vi "getFileSystem.vi"(8 "error in (no error)":errorcluster, 10 "computer":string, 11 "FileSystem in":refnum<class "FileSystem.lvclass">) -> (0 "error out":errorcluster, 3 "FileSystem out":refnum<class "FileSystem.lvclass">)   [LabVIEW 2009, in "Tools.lvlib" / "Filing.lvlib" / "FileSystem.lvclass"]
uses:
  FileSystem.lvclass
  FileSystem.lvclass/FileSystem.ctl
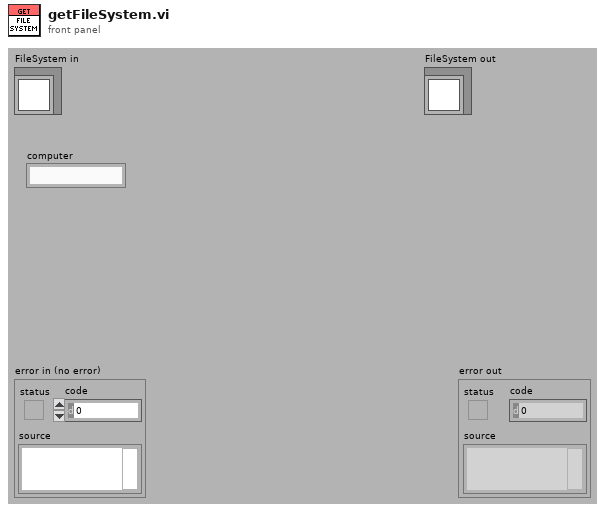
[diagram p1: front panel]
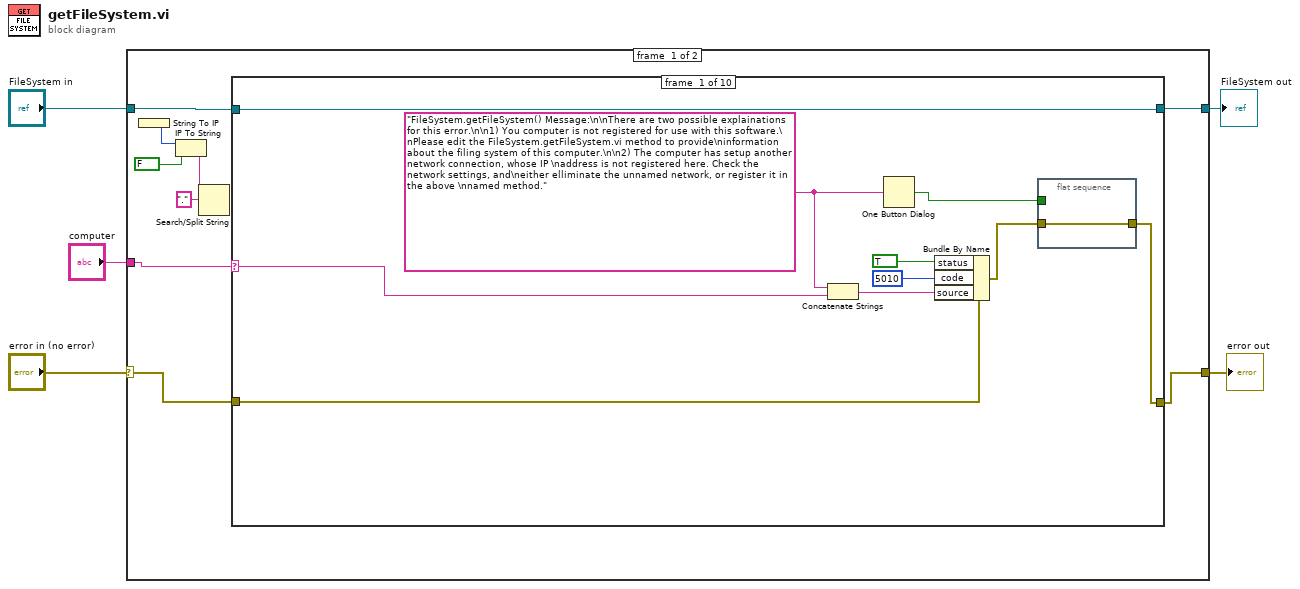
[diagram p0: block diagram]
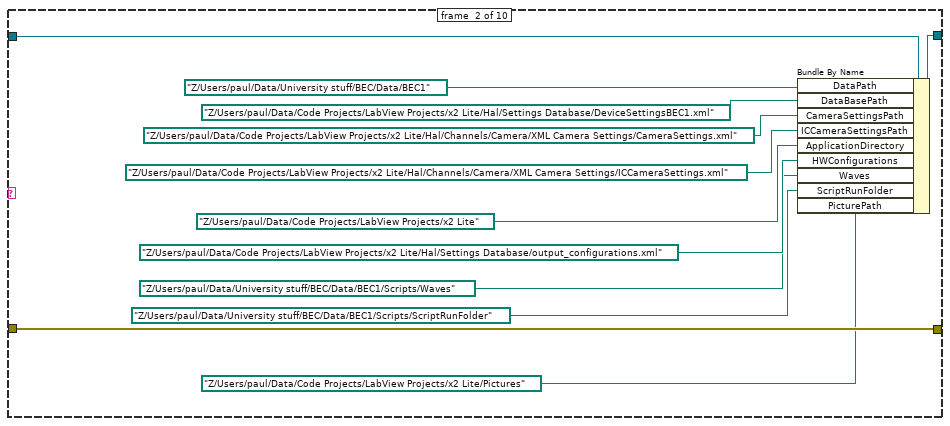
[diagram p2: hidden frame]
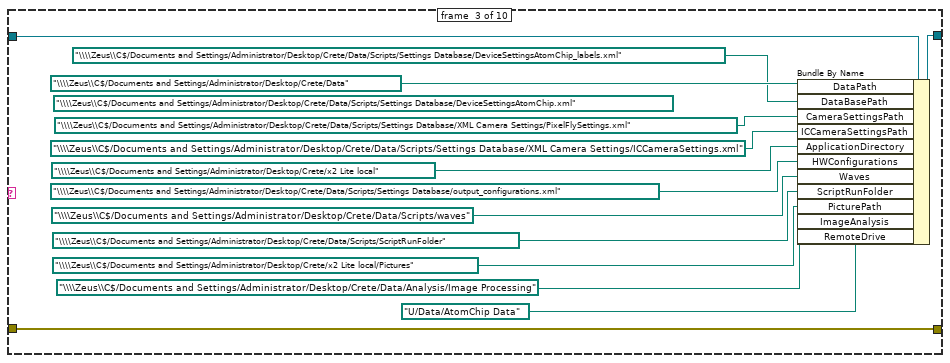
[diagram p3: hidden frame]
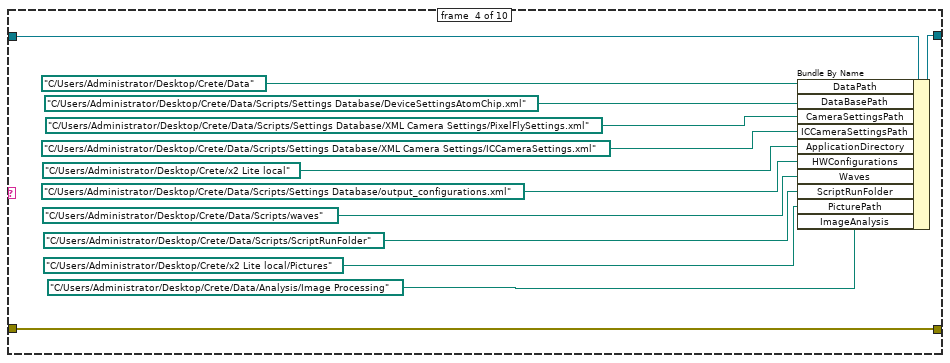
[diagram p4: hidden frame]
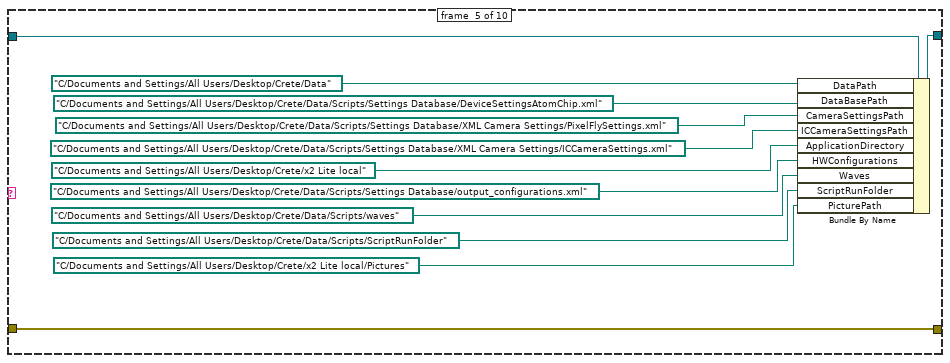
[diagram p5: hidden frame]
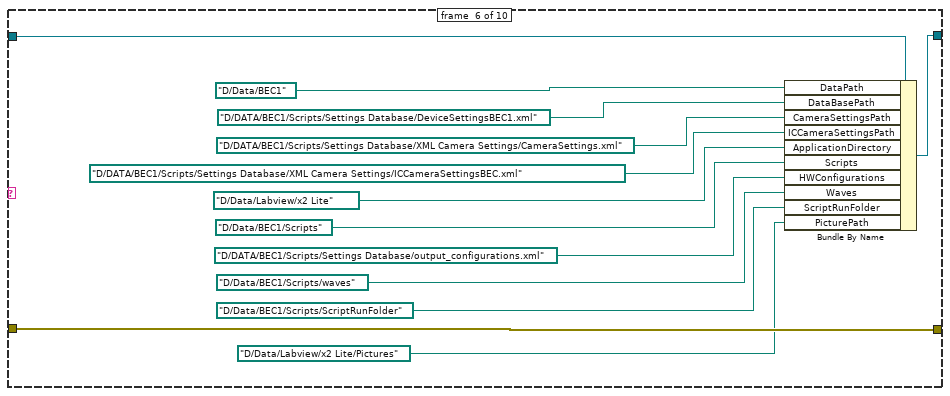
[diagram p6: hidden frame]
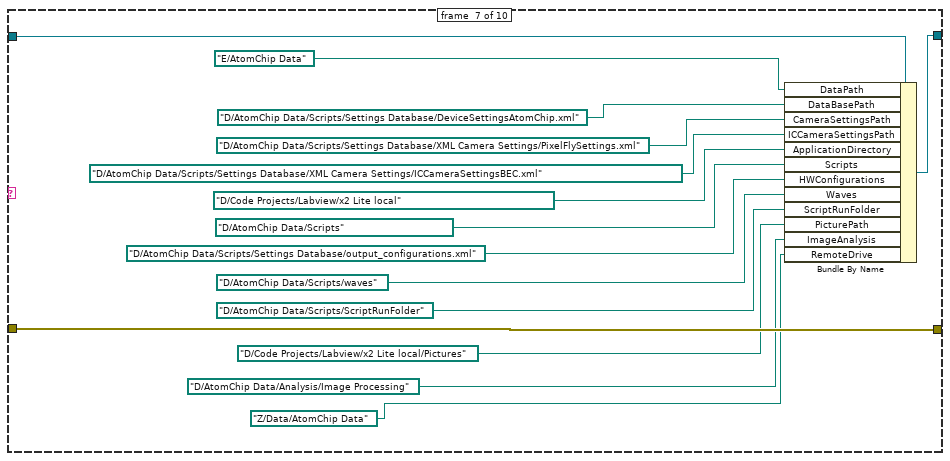
[diagram p7: hidden frame]
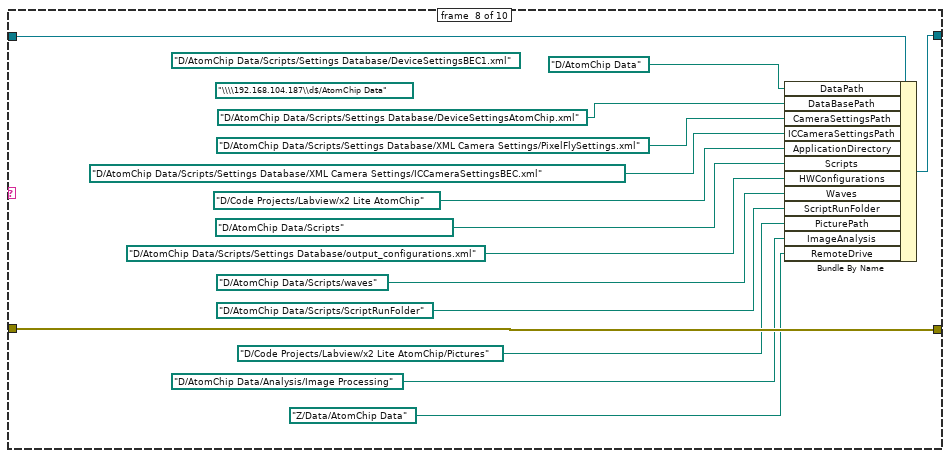
[diagram p8: hidden frame]
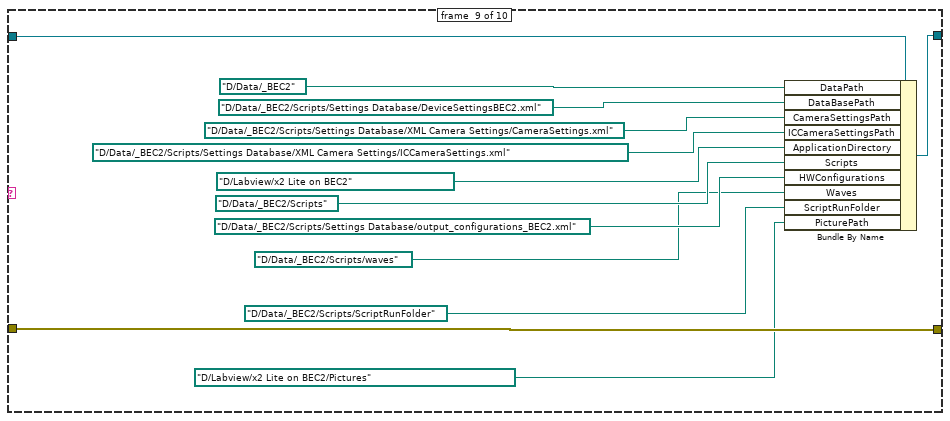
[diagram p9: hidden frame]
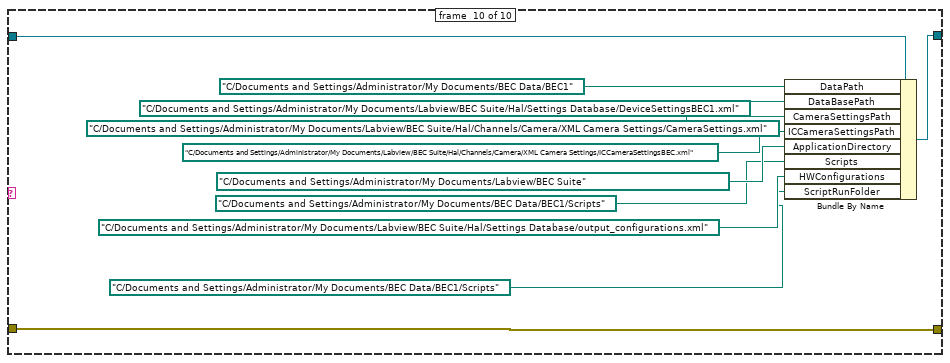
[diagram p10: hidden frame]
diagram:
  n1 = case shown="No Error" "error in (no error)" {
    selector: "error in (no error)" -> [w10 w145]
    tunnel: [w9 w145] -> w4
    tunnel: [w11 w144] -> w2
    tunnel: "FileSystem in" -> [w12 w144]
    tunnel: "computer" -> [w6 _]
    frame #0 {
      n2 = String To IP() -> (0:w13:u32)  [unwired: 1 in]
      n3 = IP To String(1:FALSE, 2:w13) -> (0:w8:string)
      n4 = Search/Split String(string=w8, search string/char (-)=".") -> ()  [unwired: 1 in, 3 out]
      n5 = case shown="\"192.168.104.187\", \"exp1\"" w6 {
        selector: w6 -> [w16 _ _ _ _ _ _ _ _ _]
        tunnel: w12 -> [w24 w37 w51 w64 w76 w89 w104 w119 w132 w143]
        tunnel: [w24 w36 w50 w63 w75 w88 w103 w118 w131 w142] -> w11
        tunnel: w10 -> [w21 w32 w47 w59 w71 w84 w100 w116 w127 w138]
        tunnel: [w19 w32 w47 w59 w71 w84 w100 w116 w127 w138] -> w9
        frame #0 {
          w17 = "FileSystem.getFileSystem() Message:\n\nThere are two possible explainations for this error.\n\n1) You computer is not registered for use with this software.\nPlease edit the FileSystem.getFileSystem.vi method to provide\ninformation about the filing system of this computer.\n\n2) The computer has setup another network connection, whose IP \naddress is not registered here. Check the network settings, and\neither elliminate the unnamed network, or register it in the above \nnamed method."
          n6 = Concatenate Strings(w17, w16) -> (w15:string)
          n7 = One Button Dialog(message=w17) -> (true=w18:bool)  [unwired: 1 in]
          n8 = Bundle By Name(cluster=w21, "status"=TRUE, "code"=5010, "source"=w15) -> (w20:errorcluster)
          n9 = flat-sequence {
            tunnel: w20 -> [w25]
            tunnel: [w25] -> w19
            tunnel: w18 -> [_]
            frame #0 {
            }
          }
        }
        frame #1 {
          n10 = Bundle By Name(cluster=w37, "DataPath"=path "Z:/Users/paul/Data/University stuff/BEC/Data/BEC1", "DataBasePath"=path "Z:/Users/paul/Data/Code Projects/LabView Projects/x2 Lite/Hal/Settings Database/DeviceSettingsBEC1.xml", "CameraSettingsPath"=path "Z:/Users/paul/Data/Code Projects/LabView Projects/x2 Lite/Hal/Channels/Camera/XML Camera Settings/CameraSettings.xml", "ICCameraSettingsPath"=path "Z:/Users/paul/Data/Code Projects/LabView Projects/x2 Lite/Hal/Channels/Camera/XML Camera Settings/ICCameraSettings.xml", "ApplicationDirectory"=path "Z:/Users/paul/Data/Code Projects/LabView Projects/x2 Lite", "HWConfigurations"=path "Z:/Users/paul/Data/Code Projects/LabView Projects/x2 Lite/Hal/Settings Database/output_configurations.xml", "Waves"=path "Z:/Users/paul/Data/University stuff/BEC/Data/BEC1/Scripts/Waves", "ScriptRunFolder"=path "Z:/Users/paul/Data/University stuff/BEC/Data/BEC1/Scripts/ScriptRunFolder", "PicturePath"=path "Z:/Users/paul/Data/Code Projects/LabView Projects/x2 Lite/Pictures") -> (w36:refnum<class "FileSystem.lvclass">)
        }
        frame #2 {
          (unwired) path "\\\\Zeus\\C$/Documents and Settings/Administrator/Desktop/Crete/Data/Scripts/Settings Database/DeviceSettingsAtomChip.xml"
          n11 = Bundle By Name(cluster=w51, "DataPath"=path "\\\\Zeus\\C$/Documents and Settings/Administrator/Desktop/Crete/Data", "DataBasePath"=path "\\\\Zeus\\C$/Documents and Settings/Administrator/Desktop/Crete/Data/Scripts/Settings Database/DeviceSettingsAtomChip_labels.xml", "CameraSettingsPath"=path "\\\\Zeus\\C$/Documents and Settings/Administrator/Desktop/Crete/Data/Scripts/Settings Database/XML Camera Settings/PixelFlySettings.xml", "ICCameraSettingsPath"=path "\\\\Zeus\\C$/Documents and Settings/Administrator/Desktop/Crete/Data/Scripts/Settings Database/XML Camera Settings/ICCameraSettings.xml", "ApplicationDirectory"=path "\\\\Zeus\\C$/Documents and Settings/Administrator/Desktop/Crete/x2 Lite local", "HWConfigurations"=path "\\\\Zeus\\C$/Documents and Settings/Administrator/Desktop/Crete/Data/Scripts/Settings Database/output_configurations.xml", "Waves"=path "\\\\Zeus\\C$/Documents and Settings/Administrator/Desktop/Crete/Data/Scripts/waves", "ScriptRunFolder"=path "\\\\Zeus\\C$/Documents and Settings/Administrator/Desktop/Crete/Data/Scripts/ScriptRunFolder", "PicturePath"=path "\\\\Zeus\\C$/Documents and Settings/Administrator/Desktop/Crete/x2 Lite local/Pictures", "ImageAnalysis"=path "\\\\Zeus\\C$/Documents and Settings/Administrator/Desktop/Crete/Data/Analysis/Image Processing", "RemoteDrive"=path "U:/Data/AtomChip Data") -> (w50:refnum<class "FileSystem.lvclass">)
        }
        frame #3 {
          n12 = Bundle By Name(cluster=w64, "DataPath"=path "C:/Users/Administrator/Desktop/Crete/Data", "DataBasePath"=path "C:/Users/Administrator/Desktop/Crete/Data/Scripts/Settings Database/DeviceSettingsAtomChip.xml", "CameraSettingsPath"=path "C:/Users/Administrator/Desktop/Crete/Data/Scripts/Settings Database/XML Camera Settings/PixelFlySettings.xml", "ICCameraSettingsPath"=path "C:/Users/Administrator/Desktop/Crete/Data/Scripts/Settings Database/XML Camera Settings/ICCameraSettings.xml", "ApplicationDirectory"=path "C:/Users/Administrator/Desktop/Crete/x2 Lite local", "HWConfigurations"=path "C:/Users/Administrator/Desktop/Crete/Data/Scripts/Settings Database/output_configurations.xml", "Waves"=path "C:/Users/Administrator/Desktop/Crete/Data/Scripts/waves", "ScriptRunFolder"=path "C:/Users/Administrator/Desktop/Crete/Data/Scripts/ScriptRunFolder", "PicturePath"=path "C:/Users/Administrator/Desktop/Crete/x2 Lite local/Pictures", "ImageAnalysis"=path "C:/Users/Administrator/Desktop/Crete/Data/Analysis/Image Processing") -> (w63:refnum<class "FileSystem.lvclass">)
        }
        frame #4 {
          n13 = Bundle By Name(cluster=w76, "DataPath"=path "C:/Documents and Settings/All Users/Desktop/Crete/Data", "DataBasePath"=path "C:/Documents and Settings/All Users/Desktop/Crete/Data/Scripts/Settings Database/DeviceSettingsAtomChip.xml", "CameraSettingsPath"=path "C:/Documents and Settings/All Users/Desktop/Crete/Data/Scripts/Settings Database/XML Camera Settings/PixelFlySettings.xml", "ICCameraSettingsPath"=path "C:/Documents and Settings/All Users/Desktop/Crete/Data/Scripts/Settings Database/XML Camera Settings/ICCameraSettings.xml", "ApplicationDirectory"=path "C:/Documents and Settings/All Users/Desktop/Crete/x2 Lite local", "HWConfigurations"=path "C:/Documents and Settings/All Users/Desktop/Crete/Data/Scripts/Settings Database/output_configurations.xml", "Waves"=path "C:/Documents and Settings/All Users/Desktop/Crete/Data/Scripts/waves", "ScriptRunFolder"=path "C:/Documents and Settings/All Users/Desktop/Crete/Data/Scripts/ScriptRunFolder", "PicturePath"=path "C:/Documents and Settings/All Users/Desktop/Crete/x2 Lite local/Pictures") -> (w75:refnum<class "FileSystem.lvclass">)
        }
        frame #5 {
          n14 = Bundle By Name(cluster=w89, "DataPath"=path "D:/Data/BEC1", "DataBasePath"=path "D:/DATA/BEC1/Scripts/Settings Database/DeviceSettingsBEC1.xml", "CameraSettingsPath"=path "D:/DATA/BEC1/Scripts/Settings Database/XML Camera Settings/CameraSettings.xml", "ICCameraSettingsPath"=path "D:/DATA/BEC1/Scripts/Settings Database/XML Camera Settings/ICCameraSettingsBEC.xml", "ApplicationDirectory"=path "D:/Data/Labview/x2 Lite", "Scripts"=path "D:/Data/BEC1/Scripts", "HWConfigurations"=path "D:/DATA/BEC1/Scripts/Settings Database/output_configurations.xml", "Waves"=path "D:/Data/BEC1/Scripts/waves", "ScriptRunFolder"=path "D:/Data/BEC1/Scripts/ScriptRunFolder", "PicturePath"=path "D:/Data/Labview/x2 Lite/Pictures") -> (w88:refnum<class "FileSystem.lvclass">)
        }
        frame #6 {
          n15 = Bundle By Name(cluster=w104, "DataPath"=path "E:/AtomChip Data", "DataBasePath"=path "D:/AtomChip Data/Scripts/Settings Database/DeviceSettingsAtomChip.xml", "CameraSettingsPath"=path "D:/AtomChip Data/Scripts/Settings Database/XML Camera Settings/PixelFlySettings.xml", "ICCameraSettingsPath"=path "D:/AtomChip Data/Scripts/Settings Database/XML Camera Settings/ICCameraSettingsBEC.xml", "ApplicationDirectory"=path "D:/Code Projects/Labview/x2 Lite local", "Scripts"=path "D:/AtomChip Data/Scripts", "HWConfigurations"=path "D:/AtomChip Data/Scripts/Settings Database/output_configurations.xml", "Waves"=path "D:/AtomChip Data/Scripts/waves", "ScriptRunFolder"=path "D:/AtomChip Data/Scripts/ScriptRunFolder", "PicturePath"=path "D:/Code Projects/Labview/x2 Lite local/Pictures", "ImageAnalysis"=path "D:/AtomChip Data/Analysis/Image Processing", "RemoteDrive"=path "Z:/Data/AtomChip Data") -> (w103:refnum<class "FileSystem.lvclass">)
        }
        frame #7 {
          (unwired) path "D:/AtomChip Data/Scripts/Settings Database/DeviceSettingsBEC1.xml"
          (unwired) path "\\\\192.168.104.187\\d$/AtomChip Data"
          n16 = Bundle By Name(cluster=w119, "DataPath"=path "D:/AtomChip Data", "DataBasePath"=path "D:/AtomChip Data/Scripts/Settings Database/DeviceSettingsAtomChip.xml", "CameraSettingsPath"=path "D:/AtomChip Data/Scripts/Settings Database/XML Camera Settings/PixelFlySettings.xml", "ICCameraSettingsPath"=path "D:/AtomChip Data/Scripts/Settings Database/XML Camera Settings/ICCameraSettingsBEC.xml", "ApplicationDirectory"=path "D:/Code Projects/Labview/x2 Lite AtomChip", "Scripts"=path "D:/AtomChip Data/Scripts", "HWConfigurations"=path "D:/AtomChip Data/Scripts/Settings Database/output_configurations.xml", "Waves"=path "D:/AtomChip Data/Scripts/waves", "ScriptRunFolder"=path "D:/AtomChip Data/Scripts/ScriptRunFolder", "PicturePath"=path "D:/Code Projects/Labview/x2 Lite AtomChip/Pictures", "ImageAnalysis"=path "D:/AtomChip Data/Analysis/Image Processing", "RemoteDrive"=path "Z:/Data/AtomChip Data") -> (w118:refnum<class "FileSystem.lvclass">)
        }
        frame #8 {
          n17 = Bundle By Name(cluster=w132, "DataPath"=path "D:/Data/_BEC2", "DataBasePath"=path "D:/Data/_BEC2/Scripts/Settings Database/DeviceSettingsBEC2.xml", "CameraSettingsPath"=path "D:/Data/_BEC2/Scripts/Settings Database/XML Camera Settings/CameraSettings.xml", "ICCameraSettingsPath"=path "D:/Data/_BEC2/Scripts/Settings Database/XML Camera Settings/ICCameraSettings.xml", "ApplicationDirectory"=path "D:/Labview/x2 Lite on BEC2", "Scripts"=path "D:/Data/_BEC2/Scripts", "HWConfigurations"=path "D:/Data/_BEC2/Scripts/Settings Database/output_configurations_BEC2.xml", "Waves"=path "D:/Data/_BEC2/Scripts/waves", "ScriptRunFolder"=path "D:/Data/_BEC2/Scripts/ScriptRunFolder", "PicturePath"=path "D:/Labview/x2 Lite on BEC2/Pictures") -> (w131:refnum<class "FileSystem.lvclass">)
        }
        frame #9 {
          n18 = Bundle By Name(cluster=w143, "DataPath"=path "C:/Documents and Settings/Administrator/My Documents/BEC Data/BEC1", "DataBasePath"=path "C:/Documents and Settings/Administrator/My Documents/Labview/BEC Suite/Hal/Settings Database/DeviceSettingsBEC1.xml", "CameraSettingsPath"=path "C:/Documents and Settings/Administrator/My Documents/Labview/BEC Suite/Hal/Channels/Camera/XML Camera Settings/CameraSettings.xml", "ICCameraSettingsPath"=path "C:/Documents and Settings/Administrator/My Documents/Labview/BEC Suite/Hal/Channels/Camera/XML Camera Settings/ICCameraSettingsBEC.xml", "ApplicationDirectory"=path "C:/Documents and Settings/Administrator/My Documents/Labview/BEC Suite", "Scripts"=path "C:/Documents and Settings/Administrator/My Documents/BEC Data/BEC1/Scripts", "HWConfigurations"=path "C:/Documents and Settings/Administrator/My Documents/Labview/BEC Suite/Hal/Settings Database/output_configurations.xml", "ScriptRunFolder"=path "C:/Documents and Settings/Administrator/My Documents/BEC Data/BEC1/Scripts") -> (w142:refnum<class "FileSystem.lvclass">)
        }
      }
    }
    frame #1 {
    }
  }
  "error out" <- w4
  "FileSystem out" <- w2
